vi "Stitch data speed image.vi"(0 "Ctrl refs":T1, 1 "Required Y-axis size of bottom tier":u32=94, 2 "Whole dataset":bool, 3 "Caller":enum16{"Viewer", "Exporter"}(ring)=enum."Exporter", 5 "Microscope image":T2, 9 "Global frame number in master video(s)":i32, 11 "error in (no error)":errorcluster, 12 "Initial frame":bool, 14 "Funct exporter":bool) -> (6 "Stitched Image":T2(plugin-control), 15 "error out":errorcluster)   [LabVIEW 2017]
uses:
  <vilib>/vision/Image Controls.llb/IMAQ Image.ctl
  Typedefs/8-bit video export window ctrl refs.ctl
  Patch-Vol video generator/Typedefs/Bright-Contr-Gamma cluster.ctl
  Typedefs/Speed graph behaviour enum.ctl
  <vilib>/vision/NI_Vision_Development_Module.lvlib
panel:
  out "Speed Chart":dbl[](graph)
  out "Bounds:Area Width":u32
  out "X Resolution":u32
  out "Image":T2(plugin-control)
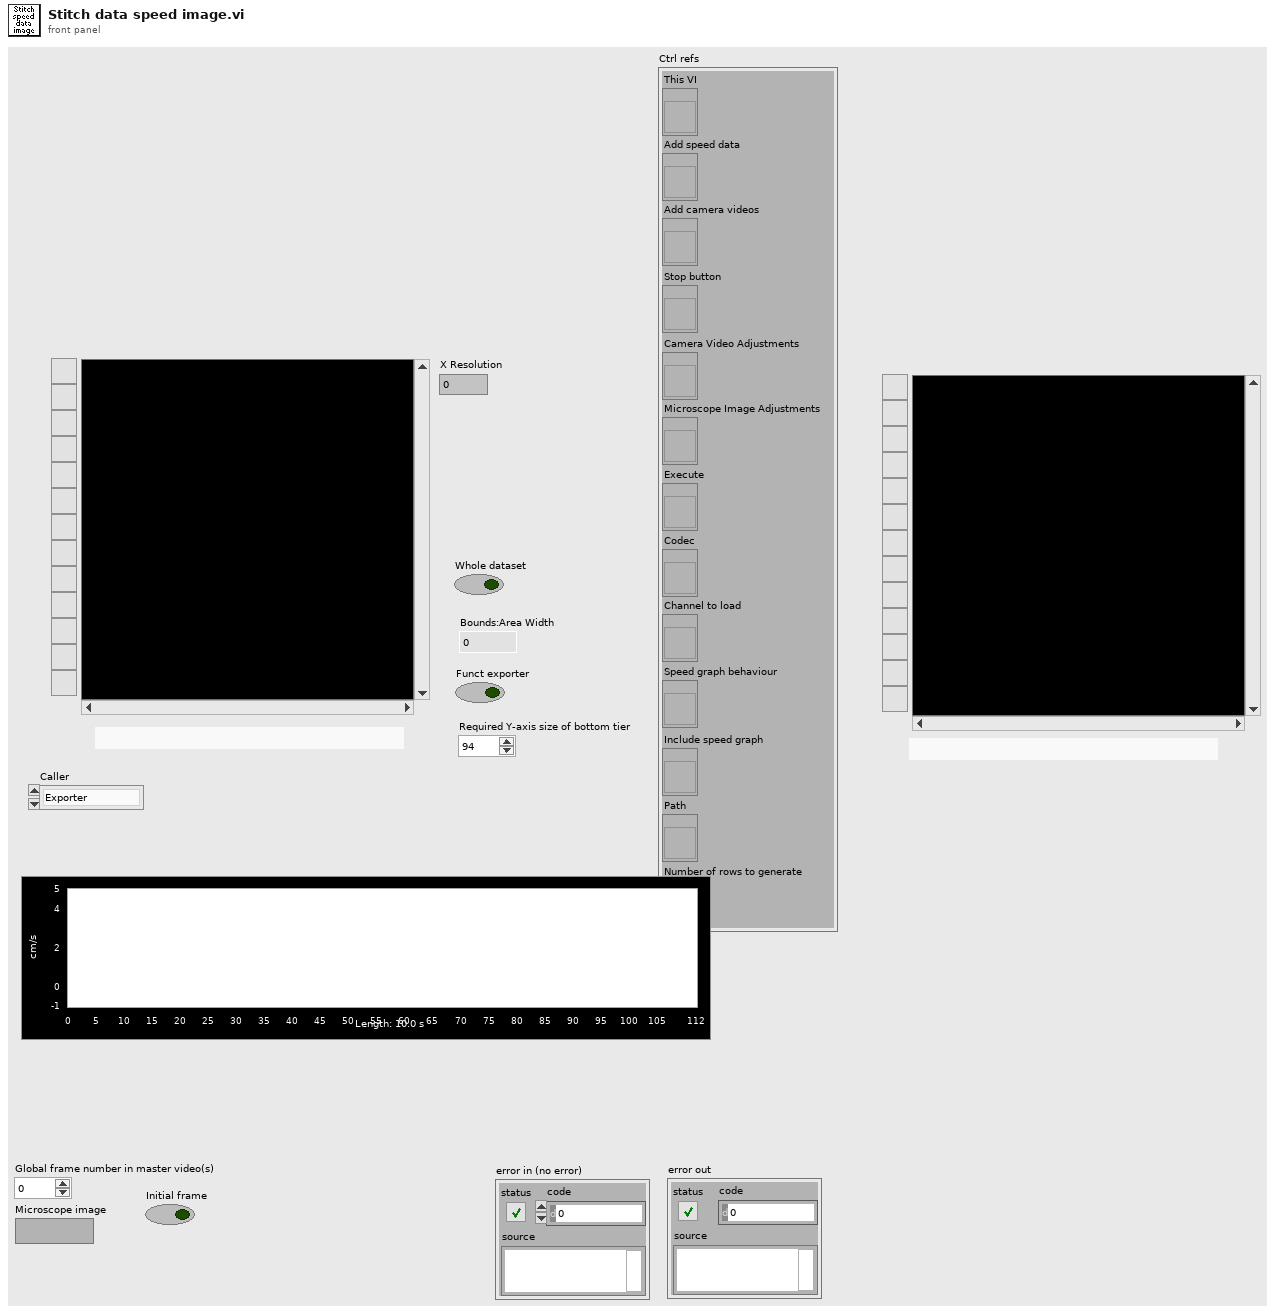
[diagram p1: front panel]
types:
  T1 = typedef "8-bit video export window ctrl refs.ctl" = cluster{"This VI":refnum<vi>, "Add speed data":refnum<vi>, "Add camera videos":refnum<vi>, "Stop button":refnum<vi>, "Camera Video Adjustments":refnum<vi>, "Microscope Image Adjustments":refnum<vi>, "Execute":refnum<vi>, "Codec":refnum<vi>, "Channel to load":refnum<vi>, "Speed graph behaviour":refnum<vi>, "Include speed graph":refnum<vi>, "Number of rows to generate":refnum<vi>, "Path":refnum<vi>}
  T2 = typedef "IMAQ Image.ctl" = refnum<image>
  T3 = typedef "Image Type" = u32
  T4 = typedef "Speed graph behaviour enum.ctl" = enum16{"Scrolling data", "Scrolling cursor"}
  T5 = typedef "imagedata.ctl" = cluster{"image type":i32, "image depth":i32, "image":u8[], "mask":u8[], "colors":u32[], "Rectangle":cluster{"left":i16, "top":i16, "right":i16, "bottom":i16}}
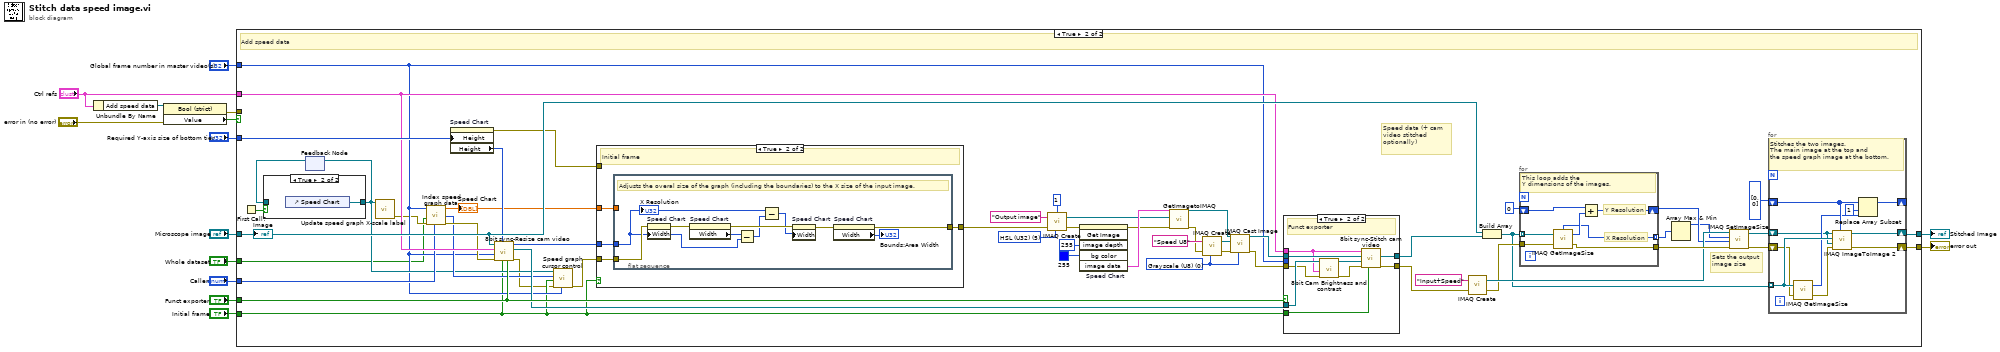
[diagram p0: block diagram]
diagram:
  n1 = Unbundle By Name("Ctrl refs") -> ("Add speed data"=w12:refnum<vi>)
  n2 = property class="Bool (strict)"(reference=w12, error in="error in (no error)") -> (error out=w9:errorcluster, "Value"=w11:bool)  [unwired: 1 out]
  n3 = case shown="True" w11 {
    tunnel: [w16 w44] -> w14
    tunnel: [w15 w43] -> w13
    tunnel: "Microscope image" -> [w16 w40]
    tunnel: w9 -> [w15 _]
    tunnel: "Initial frame" -> [_ w21]
    tunnel: "Global frame number in master video(s)" -> [_ w22]
    tunnel: "Required Y-axis size of bottom tier" -> [_ w33]
    tunnel: "Ctrl refs" -> [_ w32]
    tunnel: "Funct exporter" -> [_ w34]
    tunnel: "Caller" -> [_ w25]
    tunnel: "Whole dataset" -> [_ w17]
    frame False {
      # "Do not add speed data"
    }
    frame True {
      w62 = T3 0 items=["Grayscale (U8)", "Grayscale (I16)", "Grayscale (SGL)", "Complex (CSG)", "RGB (U32)", "HSL (U32)", "RGB (U64)", "Grayscale (U16)"] ("Image Type")
      w70 = T3 5 items=["Grayscale (U8)", "Grayscale (I16)", "Grayscale (SGL)", "Complex (CSG)", "RGB (U32)", "HSL (U32)", "RGB (U64)", "Grayscale (U16)"] ("Image Type")
      # "Speed data (+ cam video stitched optionally)"
      # "Sets the output image size"
      # "Add speed data"
      n4 = First Call?() -> (First Call?: T/F=w42:bool)
      n5 = feedback #1() -> (w41:refnum<vi>)  [unwired: 1 in]
      n6 = case shown="True" w42 {
        tunnel: [w83 w84] -> w23
        tunnel: w41 -> [w83 _]
        frame False {
        }
        frame True {
          n7 = control-ref of="Speed Chart"() -> (w84:refnum<vi>)
        }
      }
      n8 = feedback-in #1(w23) -> ()
      n9 = call "Update speed graph X-scale label.vi"("Speed Graph"=w23) -> ("error out"=w18:errorcluster)  [unwired: 10 in]
      n10 = call "Index speed graph data.vi"("Caller"=w25, "error in (no error)"=w18, "Whole dataset (F)"=w17, "Gobal frame number in Timelapse data/master video (1 based)"=w22) -> ("error out"=w27:errorcluster, "Speed data waveform graph"=w26:dbl[], "Speed graph behaviour"=w24:T4)  [unwired: 5 in]
      "Speed Chart" <- w26
      n11 = property on="Speed Chart" class="WFGraph (strict)"("Height"=w33) -> (error out=w28:errorcluster, "Height"=w30:u32)  [unwired: 2 in, 1 out]
      n12 = call "8bit sync-Resize cam video.vi"("Funct exporter"=w34, "Initial frame"=w21, "Required cam video height"=w30, "error in (no error)"=w27, "Frame number (unity based)"=w22, "Ctrl refs"=w32, "Microscope image"=w40) -> ("error out"=w20:errorcluster, "Resampled Cam video"=w29:T2, "X Resolution of speed graph"=w31:u32)  [unwired: 2 in]
      n13 = call "Speed graph cursor control.vi"("Frame number"=w22, "error in (no error)"=w20, "Initial frame"=w21, "Speed graph behaviour"=w24, "Speed graph ref"=w23) -> ("error out"=w19:errorcluster)  [unwired: 6 in]
      n14 = case shown="True" w21 {
        tunnel: w19 -> [w85 w89]
        tunnel: [w85 w88] -> w35
        tunnel: w26 -> [_ w86]
        tunnel: w31 -> [_ w87]
        tunnel: w28 -> [_ _]
        frame False {
          # "Is not the initial frame"
        }
        frame True {
          # "Initial frame"
          n15 = flat-sequence {
            tunnel: w89 -> [w91]
            tunnel: [w92] -> w88
            tunnel: w87 -> [w90]
            tunnel: w86 -> [_]
            frame #0 {
              # "Adjusts the overal size of the graph (including the boundaries) to the X size of the input image."
              n16 = property on="Speed Chart" class="WFGraph (strict)"(error in=w91, "Width"=w90) -> (error out=w94:errorcluster)  [unwired: 1 in, 1 out]
              n17 = property on="Speed Chart" class="WFGraph (strict)"(error in=w94) -> (error out=w98:errorcluster, "Width"=w99:u32)  [unwired: 1 in, 1 out]
              n18 = Subtract(x=w99, y=w90) -> (x-y=w97:u32)
              n19 = Subtract(x=w90, y=w97) -> (x-y=w96:u32)
              n20 = property on="Speed Chart" class="WFGraph (strict)"(error in=w98, "Width"=w96) -> (error out=w95:errorcluster)  [unwired: 1 in, 1 out]
              n21 = property on="Speed Chart" class="WFGraph (strict)"(error in=w95) -> (error out=w92:errorcluster, "Width"=→"Bounds:Area Width":u32)  [unwired: 1 in, 1 out]
              "X Resolution" <- w90
            }
          }
        }
      }
      n22 = call "IMAQ Create"("Border Size"=1, "Image Name"="Output image", "Image Type"=w70, "error in (no error)"=w35) -> ("New Image"=w68:T2, "error out"=w49:errorcluster)  [unwired: 1 in]
      n23 = invoke on="Speed Chart" class="WFGraph (strict)" method="Get Image"(error in=w49, "image depth"=255 ("Image Depth"), "bg color"=u32 255) -> (error out=w50:errorcluster, "image data"=w71:T5)  [unwired: 3 in, 4 out]
      n24 = call "GetImagetoIMAQ.vi"("error in (no error)"=w50, "Image Src"=w68, "Image Data"=w71) -> ("error out"=w52:errorcluster, "Image Out"=w54:T2)  [unwired: 7 in]
      n25 = call "IMAQ Create"("Image Name"="Speed U8", "Image Type"=w62, "error in (no error)"=w52) -> ("New Image"=w63:T2, "error out"=w51:errorcluster)  [unwired: 2 in]
      n26 = call "IMAQ Cast Image"("Image Type"=w62, "error in (no error)"=w51, "Image Dst"=w63, "Image Src"=w54) -> ("error out"=w39:errorcluster, "Image Dst Out"=w37:T2)  [unwired: 6 in]
      n27 = case shown="True" w34 {
        tunnel: w39 -> [w72 w74]
        tunnel: [w72 w79] -> w38
        tunnel: w32 -> [_ w76]
        tunnel: w21 -> [_ w81]
        tunnel: w22 -> [_ _]
        tunnel: w37 -> [w73 w82]
        tunnel: [w73 w80] -> w36
        tunnel: w29 -> [_ w77]
        frame False {
          # "Timelapse exporter"
        }
        frame True {
          # "Funct exporter"
          n28 = call "8bit Cam Brightness and contrast.vi"("error in (no error)"=w74, "Ctrl refs"=w76, "8bit Input image"=w77) -> ("error out"=w75:errorcluster, "8bit Output image"=w78:T2)  [unwired: 7 in]
          n29 = call "8bit sync-Stitch cam video.vi"("Initial frame"=w81, "error in (no error)"=w75, "Resampled Cam video"=w78, "Input image"=w82, "Ctrl refs"=w76) -> ("error out"=w79:errorcluster, "Output image"=w80:T2)  [unwired: 5 in]
        }
      }
      n30 = call "IMAQ Create"("Image Name"="Input+Speed", "error in (no error)"=w38) -> ("New Image"=w56:T2, "error out"=w53:errorcluster)  [unwired: 2 in, 1 out]
      n31 = Build Array(w40, w36) -> (w48:T2[])
      n32 = for {
        tunnel: w48 -> [w116] mode=indexing
        shift-right: [w114] -> w47
        shift-left: 0 ("Y Resolution") -> [w115]
        tunnel: [w110] -> w46 mode=indexing
        tunnel: [w113] -> w59
        tunnel: w53 -> [w112]
        # "Y Resolution"
        # "X Resolution"
        # "This loop adds the \nY dimensions of the images."
        n33 = call "IMAQ GetImageSize"("Image"=w116, "error in (no error)"=w112) -> ("Y Resolution"=w111:i32, "X Resolution"=w110:i32, "error out"=w113:errorcluster)  [unwired: 2 out]
        n34 = Add(x=w115, y=w111) -> (x+y=w114:i32)
      }
      n35 = Array Max & Min(array=w46) -> (max value=w45:i32)  [unwired: 3 out]
      n36 = call "IMAQ SetImageSize"("error in (no error)"=w59, "Y Resolution"=w47, "X Resolution"=w45, "Image"=w56) -> ("error out"=w58:errorcluster, "Image Out"=w55:T2)  [unwired: 1 out]
      n37 = for {
        tunnel: w48 -> [w109] mode=indexing
        shift-right: [w108] -> _
        shift-left: i32[] [0, 0] -> [w107]
        shift-right: [w104] -> w44
        shift-left: w55 -> [w102]
        shift-right: [w100] -> w43
        shift-left: w58 -> [w101]
        # "Stitches the two images.\nThe main image at the top and \nthe speed graph image at the bottom."
        n38 = call "IMAQ GetImageSize"("Image"=w109, "error in (no error)"=w101) -> ("Y Resolution"=w105:i32, "error out"=w103:errorcluster)  [unwired: 3 out]
        n39 = call "IMAQ ImageToImage 2"("Offset Left/Top"=w107, "error in (no error)"=w103, "Image Dst"=w102, "Image Src (Small)"=w109, "Image Src (Large)"=w102) -> ("error out"=w100:errorcluster, "Image Dst Out"=w104:T2)  [unwired: 1 in, 4 out]
        n40 = Replace Array Subset(array=w107, new element=w105, index=1) -> (w108:i32[])
      }
      "Image" <- w40
    }
  }
  "Stitched Image" <- w14
  "error out" <- w13
